vi "Drive Sideways.vi"(8 "error in (no error)":errorcluster, 10 "Joystick State":cluster{"Buttons":T1[], "Axis":T2[]}, 11 "Driver in":refnum<class "Driver.lvclass">) -> (0 "error out":errorcluster, 3 "Driver out":refnum<class "Driver.lvclass">)   [LabVIEW 2014, in "Driver.lvlib" / "Driver.lvclass"]
uses:
  Driver.lvclass
  Joystick/Joystick Class/Button State.ctl
  Joystick/Joystick Class/Axis State.ctl
  Driver.lvclass/Driver.ctl
  Sideways Drive/Sideways Drive Messages/Set Percentage Msg/Set Percentage Msg.lvclass/Set Percentage Msg.ctl
  <vilib>/ActorFramework/Message Enqueuer/Message Enqueuer.lvclass/Message Enqueuer.ctl
  <vilib>/ActorFramework/Message Enqueuer/Enqueue.vi
  <vilib>/ActorFramework/Message Priority Queue/Priority Enqueue.vi
  Sideways Drive/Sideways Drive Messages/Set Percentage Msg/Set Percentage Msg.lvclass
  Joystick/Joystick.lvlib
  Joystick/Joystick Class/Joystick.lvclass
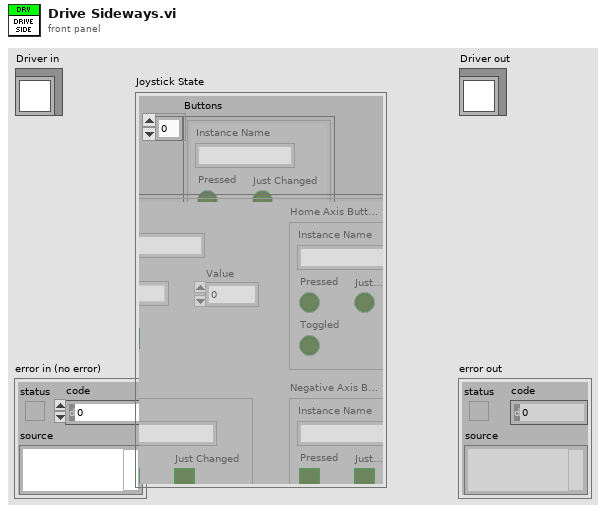
[diagram p1: front panel]
types:
  T1 = typedef "Joystick.lvlib/Joystick.lvclass/Button State.ctl" = cluster{"Pressed":bool, "Instance Name":string, "Toggled":bool, "Just Changed":bool}
  T2 = typedef "Joystick.lvlib/Joystick.lvclass/Axis State.ctl" = cluster{"Instance Name":string, "Deadband":dbl, "Value":dbl, "At Home":bool, "Postive Axis Button State":T1, "Negative Axis Button State":T1, "Home Axis Button State":T1}
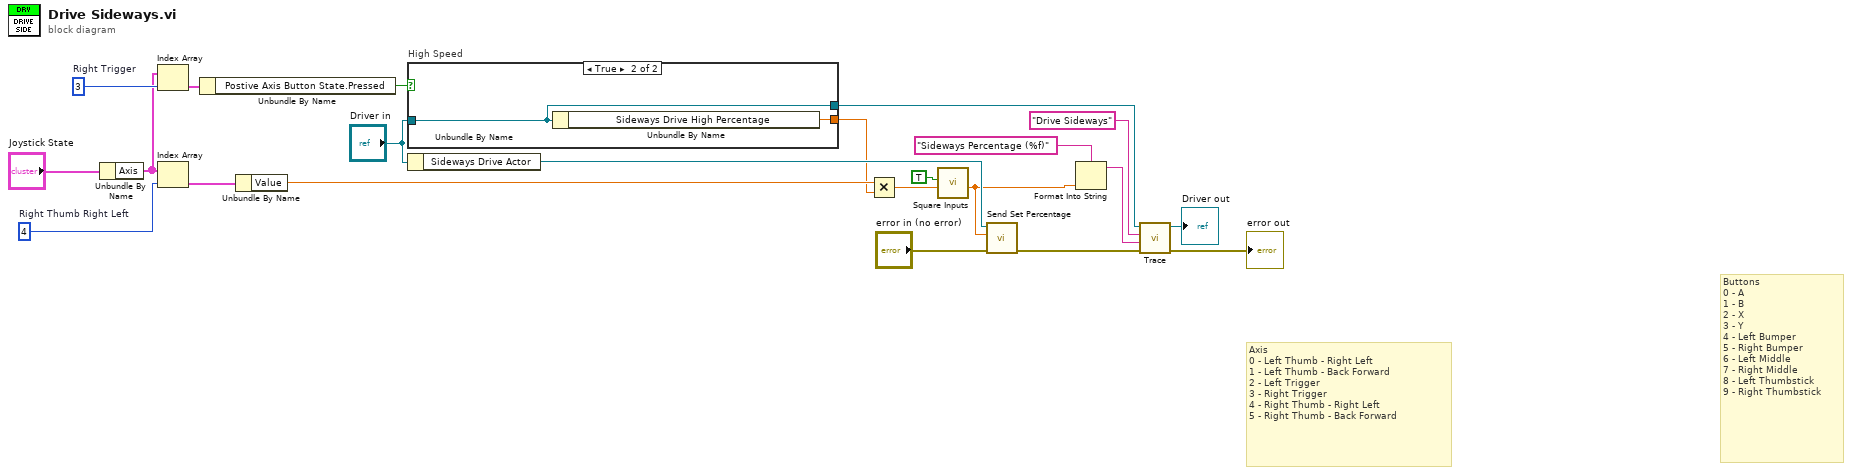
[diagram p0: block diagram]
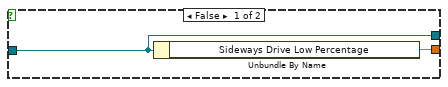
[diagram p2: hidden frame]
diagram:
  w7 = 3  # Right Trigger
  w18 = 4  # Right Thumb Right Left
  # "Buttons\n0 - A\n1 - B\n2 - X\n3 - Y\n4 - Left Bumper\n5 - Right Bumper\n6 - Left Middle\n7 - Right Middle\n8 - Left Thumbstick\n9 - Right Thumbstick"
  # "Axis\n0 - Left Thumb - Right Left\n1 - Left Thumb - Back Forward\n2 - Left Trigger\n3 - Right Trigger\n4 - Right Thumb - Right Left\n5 - Right Thumb - Back Forward"
  n1 = Unbundle By Name("Joystick State") -> ("Axis"=w6:T2[])
  n2 = Index Array(array=w6, index=w7) -> (element=w5:T2)
  n3 = Index Array(array=w6, index=w18) -> (element=w17:T2)
  n4 = Unbundle By Name(w5) -> ("Postive Axis Button State.Pressed"=w4:bool)
  n5 = Unbundle By Name(w17) -> ("Value"=w16:dbl)
  n6 = case "High Speed" shown="True" w4 {
    tunnel: "Driver in" -> [w24 w26]
    tunnel: [w24 w26] -> w2
    tunnel: [w23 w25] -> w1
    frame False {
      n7 = Unbundle By Name(w24) -> ("Sideways Drive Low Percentage"=w23:dbl)
    }
    frame True {
      n8 = Unbundle By Name(w26) -> ("Sideways Drive High Percentage"=w25:dbl)
    }
  }
  n9 = Unbundle By Name("Driver in") -> ("Sideways Drive Actor"=w12:refnum<class "Message Enqueuer.lvclass">)
  n10 = Multiply(x=w16, y=w1) -> (x*y=w10:dbl)
  n11 = call "Square Inputs.vi"("Before Square"=w10, "Square Inputs"=TRUE) -> ("After Square"=w11:dbl)  [unwired: 9 in]
  n12 = call "Send Set Percentage.vi"("error in (no error)"="error in (no error)", "Sideways Motors Percentage"=w11, "Message Enqueuer"=w12) -> ("error out"=w8:errorcluster)  [unwired: 7 in, 1 out]
  n13 = Format Into String(format string="Sideways Percentage (%f)", w11) -> (resulting string=w9:string)  [unwired: 2 in, 1 out]
  n14 = call-dynamic "Trace.vi"("error in (no error)"=w8, "System Message"=w9, "System Action"="Drive Sideways", "System Actor in"=w2) -> ("error out"=→"error out":errorcluster, "System Actor out"=→"Driver out":refnum<class "Driver.lvclass">)  [unwired: 6 in]
